vi "Report_Do.vi"(8 "error in (no error)":errorcluster, 10 "Project Builder in":refnum<class "Project Builder.lvclass">, 11 "Report Action in":refnum<class "Report Action.lvclass">) -> (0 "error out":errorcluster)   [LabVIEW 2019, in "ProjectBuilder.lvlib" / "Report Action.lvclass"]
doc: "Perform a report action. Report data and report folder path can be extracted from the Project Builder.\n\nThe default implementation does nothing."
uses:
  Report Action.lvclass
  Project Builder/Project Builder.lvclass
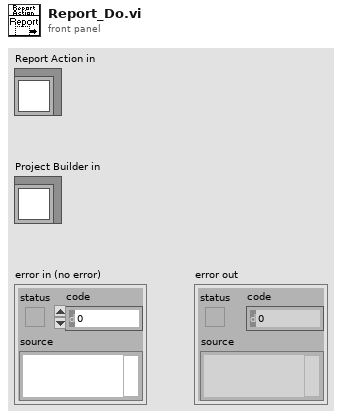
[diagram p1: front panel]
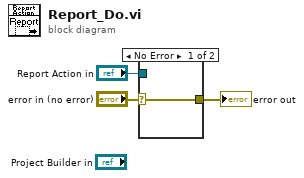
[diagram p0: block diagram]
diagram:
  n1 = case shown="No Error" "error in (no error)" {
    selector: "error in (no error)" -> [w4 w5]
    tunnel: [w4 w5] -> w2
    tunnel: "Report Action in" -> [_ _]
    frame No Error {
    }
    frame Error {
    }
  }
  "error out" <- w2
